vi "Pack for gRPC.vi"(8 "error in (no error)":errorcluster, 9 "Configuration / Resuls (Config)":enum16{"Configuration", "Results"}(ring), 10 "Data Value":variant, 11 "Measurement Customizations in":refnum<class "MeasurementPlugin.lvclass">) -> (0 "error out":errorcluster, 2 "Any":T1, 3 "Measurement Customizations out":refnum<class "MeasurementPlugin.lvclass">)   [LabVIEW 2022 SP3, in "Noise Sweep_Class D Amplifier.lvlib" / "MeasurementPlugin.lvclass"]
uses:
  MeasurementPlugin.lvclass
  MeasurementPlugin.lvclass/MeasurementPlugin.ctl
  Measurement Configuration.ctl
  Noise Sweep_Class D Amplifier.lvlib
  Measurement Results.ctl
  a6012965-5700-4384-8228-972e71b6560c.vi
  2eca732d-dbaa-43bf-a7dd-ede2da65bc1b.vi
  shared/controls/weighting filter.ctl
  shared/DAQmx/input terminal configuration.ctl
  shared/DAQmx/DAQmx utility.lvlib
  shared/controls/highpass filter.ctl
  shared/controls/lowpass filter.ctl
  <vilib>/Plug-In SDKs/Measurements/Measurement Plugin Service/Measurement Plugin Service.lvclass
  C:/Program Files/National Instruments/LabVIEW 2022/vi.lib/Plug-In SDKs/Measurements/Measurement Plugin Service/Measurement Plugin Service.lvclass
  C:/dev/class-d-amplifier/source/noise sweep/Noise Sweep_Class D Amplifier/Advanced/MeasurementPlugin.lvclass
  <vilib>/gRPC/LabVIEW gRPC Library/Shared/Any.ctl
  <vilib>/gRPC/LabVIEW gRPC Library/grpc-lvsupport-release.lvlib
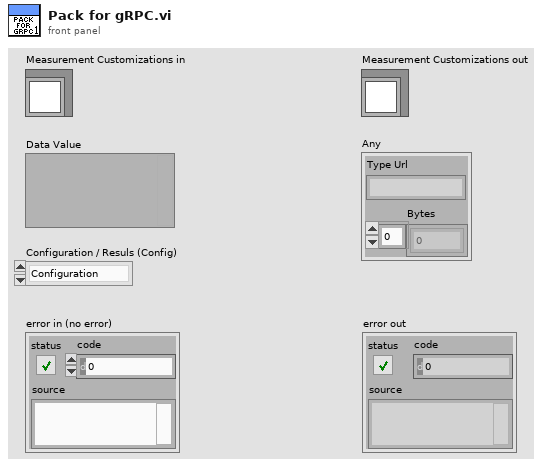
[diagram p1: front panel]
types:
  T1 = typedef "grpc-lvsupport-release.lvlib/Any.ctl" = cluster{"Type Url":string, "Bytes":u8[]}
  T2 = typedef "grpc-lvsupport-release.lvlib/grpcId.ctl" = u64
  T3 = typedef "Noise Sweep_Class D Amplifier.lvlib/Measurement Configuration.ctl" = cluster{"digital serial cfg file":string, "digital channel list":string, "master clock channel list":string, "acq channel":string, "acq sampling rate":dbl, "measurement time (s)":dbl, "delay before measurement (s)":dbl, "input range":dbl, "input terminal cfg":T4, "weighting filter":T5, "lowpass filter":T6, "highpass filter":T7, "power supply resource":string, "power supply voltage start":dbl, "power supply voltage stop":dbl, "sweep number of steps":u32, "power supply current limit":dbl}
  T4 = typedef "DAQmx utility.lvlib/input terminal configuration.ctl" = enum32{"Default", "NRSE", "RSE", "Differential", "Pseudodifferential"}
  T5 = typedef "weighting filter.ctl" = enum32{"Linear", "A-weighting", "B-weighting", "C-weighting"}
  T6 = typedef "lowpass filter.ctl" = enum32{"No filter", "AES17 20kHz", "AES17 40kHz"}
  T7 = typedef "highpass filter.ctl" = enum32{"DC", "AC"}
  T8 = typedef "Noise Sweep_Class D Amplifier.lvlib/Measurement Results.ctl" = cluster{"channel names":string[], "power supply voltage (V)":dbl[], "idle channel noise (Vrms)":dbl[], "wfm - dt":dbl, "wfm - data":dbl[]}
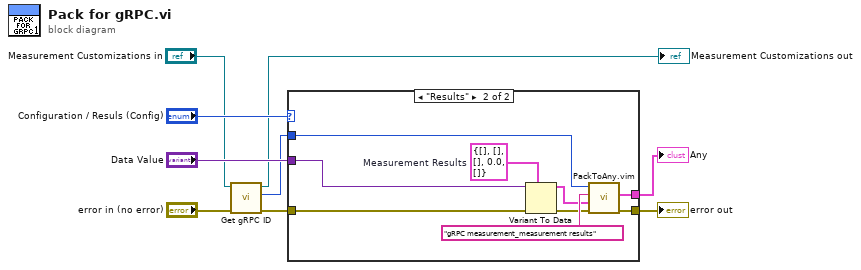
[diagram p0: block diagram]
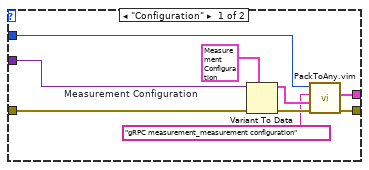
[diagram p2: hidden frame]
diagram:
  n1 = call <vilib>:"Get gRPC ID.vi"("error in"="error in (no error)", "measurement plugin service in"="Measurement Customizations in") -> ("error out"=w4:errorcluster, "gRPC ID"=w1:T2, "measurement plugin service out"=→"Measurement Customizations out":refnum<class "MeasurementPlugin.lvclass">)  [unwired: 7 in]
  n2 = case shown="\"Results\"" "Configuration / Resuls (Config)" {
    tunnel: w4 -> [w18 w27]
    tunnel: "Data Value" -> [w17 w26]
    tunnel: w1 -> [w14 w22]
    tunnel: [w16 w24] -> w8
    tunnel: [w15 w23] -> w7
    frame "Configuration" {
      w11 = T3 {"digital serial cfg file"="", "digital channel list"="7821\\PCMo 8", "master clock channel list"="7821\\PCMo 0", "acq channel"="", "acq sampling rate"=1000.0, "measurement time (s)"=0.0, "delay before measurement (s)"=0.1, "input range"=5.0, "input terminal cfg"=enum."Default", "weighting filter"=enum."Linear", "lowpass filter"=enum."No filter", "highpass filter"=enum."DC", "power supply resource"="", "power supply voltage start"=20.0, "power supply voltage stop"=20000.0, "sweep number of steps"=1, "power supply current limit"=0.0}  # Measurement Configuration
      n3 = Variant To Data(error in=w18, type=w11, Variant=w17) -> (data=w13:T3, error out=w12:errorcluster)
      n4 = call "PackToAny.vim"("error in"=w12, "Data To Pack"=w13, "Message Type"="gRPC measurement_measurement configuration", "gRPCid in"=w14) -> ("error out"=w16:errorcluster, "Any"=w15:T1)  [unwired: 5 in, 1 out]
    }
    frame "Results" {
      w25 = T8 {"channel names"=[], "power supply voltage (V)"=[], "idle channel noise (Vrms)"=[], "wfm - dt"=0.0, "wfm - data"=[]}  # Measurement Results
      n5 = Variant To Data(error in=w27, type=w25, Variant=w26) -> (data=w20:T8, error out=w19:errorcluster)
      n6 = call "PackToAny.vim"("error in"=w19, "Data To Pack"=w20, "Message Type"="gRPC measurement_measurement results", "gRPCid in"=w22) -> ("error out"=w24:errorcluster, "Any"=w23:T1)  [unwired: 5 in, 1 out]
    }
  }
  "error out" <- w8
  "Any" <- w7
